vi "SetConfigurationString.vi"(8 "ErrorIn":errorcluster, 9 "String":string, 10 "Identification":string, 11 "ReferenceIn":refnum<class "AppConfigJSON.lvclass">) -> (0 "ErrorOut":errorcluster, 3 "ReferenceOut":refnum<class "AppConfigJSON.lvclass">)   [LabVIEW 2021, in "AppConfigJSON.lvclass"]
uses:
  AppConfigJSON.lvclass
  AppConfigJSON.lvclass/AppConfigJSON.ctl
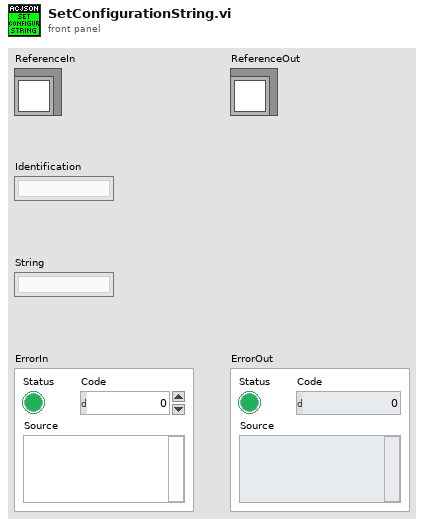
[diagram p1: front panel]
types:
  T1 = typedef "AppConfigJSON.lvclass/ObjectAttributes.ctl" = cluster{"Name":string, "ConfigFilePath":path, "Objects":T2[], "ApplicationBasePath":path, "ObjectName":string}
  T2 = typedef "IApplicationConfiguration.lvclass/ObjectDataDetails.ctl" = cluster{"ObjectName":string, "ObjectType":string, "Interfaces":T3[]}
  T3 = typedef "IApplicationConfiguration.lvclass/ObjectData.ctl" = cluster{"Label":string, "ObjectName":string, "Type":string}
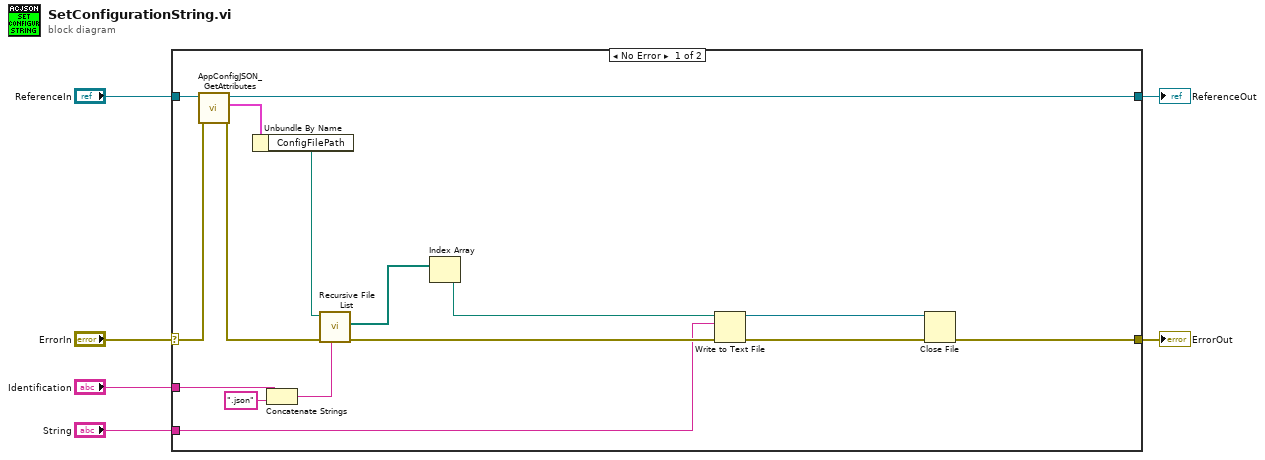
[diagram p0: block diagram]
diagram:
  n1 = case shown="No Error" "ErrorIn" {
    selector: "ErrorIn" -> [w21 w23]
    tunnel: [w18 w23] -> w5
    tunnel: [w15 w22] -> w3
    tunnel: "ReferenceIn" -> [w16 w22]
    tunnel: "Identification" -> [w13 _]
    tunnel: "String" -> [w9 _]
    frame No Error {
      n2 = call "AppConfigJSON_GetAttributes.vi"("ErrorIn"=w21, "ReferenceIn"=w16) -> ("ErrorOut"=w20:errorcluster, "Data"=w17:T1, "ReferenceOut"=w15:refnum<class "AppConfigJSON.lvclass">)  [unwired: 6 in, 1 out]
      n3 = Unbundle By Name(w17) -> ("ConfigFilePath"=w14:path)
      n4 = Concatenate Strings(w13, ".json" ("string")) -> (w11:string)
      n5 = call <vilib>:"Recursive File List.vi"("pattern"=w11, "error in (no error)"=w20, "Folder Path"=w14) -> ("All Files in Dir"=w10:path[])  [unwired: 4 in, 4 out]
      n6 = Index Array(array=w10) -> (element=w8:path)  [unwired: 1 in]
      n7 = Write to Text File(file (use dialog)=w8, text=w9, error in=w20) -> (refnum out=w7:refnum<file>, error out=w19:errorcluster)  [unwired: 1 in, 1 out]
      n8 = Close File(refnum=w7, error in=w19) -> (error out=w18:errorcluster)  [unwired: 1 out]
    }
    frame Error {
    }
  }
  "ErrorOut" <- w5
  "ReferenceOut" <- w3
